vi "auto_calc.vi"(9 "Elapsed Seconds":dbl) -> (3 "Outputs":T1)   [LabVIEW 2013]
uses:
  outputs.ctl
  drive/drive_outputs.ctl
  flinger/flinger_outputs.ctl
  <vilib>/Rock Robotics/WPI/Solenoid/WPI_SolenoidValue.ctl
  roller/roller_outputs.ctl
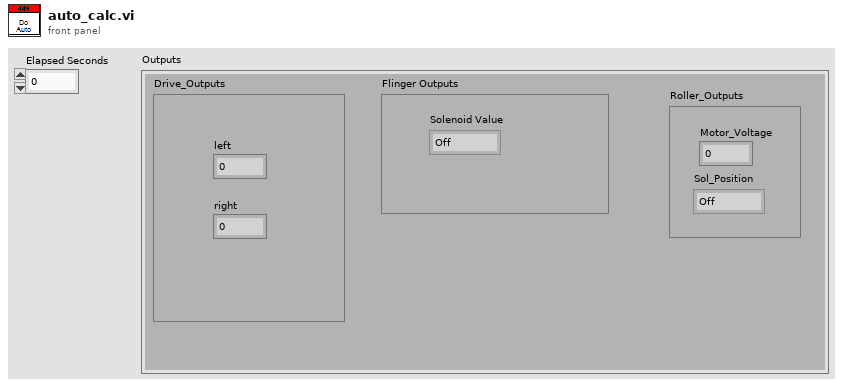
[diagram p1: front panel]
types:
  T1 = typedef "outputs.ctl" = cluster{"Drive_Outputs":T2, "Flinger Outputs":T3, "Roller_Outputs":T5}
  T2 = typedef "drive_outputs.ctl" = cluster{"left":dbl, "right":dbl}
  T3 = typedef "flinger_outputs.ctl" = cluster{"Solenoid Value":T4}
  T4 = typedef "WPI_SolenoidValue.ctl" = enum16{"Off", "On", "Forward", "Reverse"}
  T5 = typedef "roller_outputs.ctl" = cluster{"Sol_Position":T4, "Motor_Voltage":dbl}
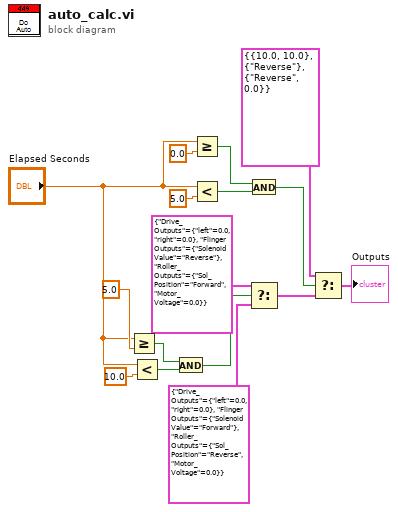
[diagram p0: block diagram]
diagram:
  n1 = Greater Or Equal?(x="Elapsed Seconds", y=5.0) -> (x >= y?=w7:bool)
  n2 = Less?(x="Elapsed Seconds", y=10.0) -> (x < y?=w6:bool)
  n3 = And(x=w7, y=w6) -> (x .and. y?=w4:bool)
  n4 = Greater Or Equal?(x="Elapsed Seconds", y=0.0) -> (x >= y?=w14:bool)
  n5 = Less?(x="Elapsed Seconds", y=5.0) -> (x < y?=w13:bool)
  n6 = And(x=w14, y=w13) -> (x .and. y?=w12:bool)
  n7 = Select(t=T1 {"Drive_Outputs"={"left"=0.0, "right"=0.0}, "Flinger Outputs"={"Solenoid Value"=enum."Reverse"}, "Roller_Outputs"={"Sol_Position"=enum."Forward", "Motor_Voltage"=0.0}} ("Outputs"), s=w4, f=T1 {"Drive_Outputs"={"left"=0.0, "right"=0.0}, "Flinger Outputs"={"Solenoid Value"=enum."Forward"}, "Roller_Outputs"={"Sol_Position"=enum."Reverse", "Motor_Voltage"=0.0}} ("Outputs")) -> (s? t:f=w2:T1)
  n8 = Select(t=T1 {"Drive_Outputs"={"left"=10.0, "right"=10.0}, "Flinger Outputs"={"Solenoid Value"=enum."Reverse"}, "Roller_Outputs"={"Sol_Position"=enum."Reverse", "Motor_Voltage"=0.0}} ("Outputs"), s=w12, f=w2) -> (s? t:f=→"Outputs":T1)
